vi "RydbergExpControl_2014.09.17_beta.vi"() -> ()   [LabVIEW 2013]
uses:
  rydberg_state_machine_states.ctl
  <userlib>/atmcd32d.llb/AcquisitionMode_mode typedef.ctl
  <userlib>/atmcd32d.llb/TriggerMode_mode typedef.ctl
  AndorCamera/camera_controls.ctl
  6704/6704_static_voltages_control.ctl
panel:
  in  "What To Change":enum16{"PulseBlaster", "Static Voltage"}(ring)
  in  "Trigger Snap Mode":bool
  in  "Shutdown Experiment":bool
  in  "Start Experiment":bool
  out "Started in trigger snap":bool=TRUE
  out "Waveform Chart":dbl(graph)
  in  "Count Number?":bool
  out "Number":dbl format="%^#_6g"
  out "OD":dbl[][](graph)
  out "Atom Closeup":dbl[][](graph)
  out "Atoms - BG":dbl[][](graph)
  out "Background Image":dbl[][](graph)
  out "Atom Image":dbl[][](graph)
  in  "Tab Control":T1(tab)
  out "Camera Ready":bool
  out "Exp Running":bool
  in  "PB Instruction Time To Change":i32
  in  "Static Channel To Change":i32
  in  "Step Size":dbl min=1e-06
  in  "Final Value":dbl
  in  "Initial Value":dbl
  in  "Instructions":T2(array[cluster])=[{"Instruct Data"=0, "Op Code"=0, "Flags"=[TRUE, FALSE, FALSE, FALSE, FALSE, FALSE, FALSE, FALSE, FALSE, FALSE, FALSE, FALSE, FALSE, FALSE, FALSE, FALSE, FALSE, FALSE, FALSE, FALSE, FALSE, FALSE, FALSE, FALSE], "Comments"="", "Time (s)"=0.1}, {"Instruct Data"=0, "Op Code"=0, "Flags"=[FALSE, FALSE, FALSE, FALSE, FALSE, FALSE, FALSE, FALSE, FALSE, FALSE, FALSE, FALSE, FALSE, FALSE, FALSE, FALSE, FALSE, FALSE, FALSE, FALSE, FALSE, FALSE, FALSE, FALSE], "Comments"="", "Time (s)"=0.1}, {"Instruct Data"=0, "Op Code"=0, "Flags"=[TRUE, FALSE, FALSE, FALSE, FALSE, FALSE, FALSE, FALSE, FALSE, FALSE, FALSE, FALSE, FALSE, FALSE, FALSE, FALSE, FALSE, FALSE, FALSE, FALSE, FALSE, FALSE, FALSE, FALSE], "Comments"="", "Time (s)"=0.1}, {"Instruct Data"=0, "Op Code"=6, "Flags"=[FALSE, FALSE, FALSE, FALSE, FALSE, FALSE, FALSE, FALSE, FALSE, FALSE, FALSE, FALSE, FALSE, FALSE, FALSE, FALSE, FALSE, FALSE, FALSE, FALSE, FALSE, FALSE, FALSE, FALSE], "Comments"="", "Time (s)"=0.1}] {"Time (s)" format="%.3p"; "Op Code" items=["Continue", "Stop", "Loop", "End Loop", "JSR", "RTS", "Branch", "Long Delay", "Wait"]}
  out "Scan Progress":dbl(slide) caption="Slide" scale=0.0..100.0
  out "Current Param Value":dbl
  in  "Parameter Nickname (no spaces)":string[](array[string])
  in  "Number of Parameters to Scan":i32=1 min=1
  in  "Channels to Change":dbl[](array[numeric])=[0.0, 0.0, 0.0]
  in  "Parameters to Change":enum16{"PulseBlaster", "Static Voltage"}[](array[ring])=[enum."Static Voltage", enum."Static Voltage", enum."Static Voltage"]
  in  "Step Sizes":dbl[](array[numeric])=[0.0, 0.0, 0.0]
  in  "Final Values":dbl[](array[numeric])=[0.0, 0.0, 0.0]
  in  "Initial Values":dbl[](array[numeric])
  in  "Scan Base Name":string
  in  "Raw_Data Folder":path
  out "Full Scan Name":string
  out "Camera Information":T3 {"VS Speed (us)" format="%.2f"}
  in  "Acquisition Parameters":T4={"Acquisition Mode"=enum."Kinetics", "Trigger Mode"=enum."External", "Frame \nTransfer"=FALSE, "Exposure Time (s)"=0.0001, "Accumulation Cycle Time (s)"=0.0, "# Accumulations"=1, "# Kinetics"=2, "Kinetic Cycle Time (s)"=0.0, "Horizontal Bin Size"=1, "Vertical Bin Size"=1} {"Vertical Bin Size" min=1; "Horizontal Bin Size" min=1; "Kinetic Cycle Time (s)" format="%.2f"; "# Kinetics" min=1; "# Accumulations" min=1; "Accumulation Cycle Time (s)" format="%.2f"; "Exposure Time (s)" format="%.2e"}
  out "Calcualted Times":T7 {"Kinetic" format="%.4f"; "Accumulate" format="%.4f"; "Exposure" format="%.4f"}
  in  "Red MOT 87 Inputs":T8={"Active Device"="6733_Red_87", "Active Channels"=[TRUE, FALSE, FALSE, FALSE, FALSE, FALSE, FALSE, FALSE], "Waveform Parameters"=[[{"Functional Form"=enum."Polynomial", "Start Voltage"=0.0, "End Voltage"=0.0, "Time"=0.0, "Degree"=1, "Sample Rate"=0.0}, {"Functional Form"=enum."Exponential", "Start Voltage"=0.0, "End Voltage"=0.0, "Time"=0.0, "Degree"=1, "Sample Rate"=0.0}, {"Functional Form"=enum."Exponential", "Start Voltage"=0.0, "End Voltage"=0.0, "Time"=0.0, "Degree"=1, "Sample Rate"=0.0}, {"Functional Form"=enum."Exponential", "Start Voltage"=0.0, "End Voltage"=0.0, "Time"=0.0, "Degree"=1, "Sample Rate"=0.0}, {"Functional Form"=enum."Exponential", "Start Voltage"=0.0, "End Voltage"=0.0, "Time"=0.0, "Degree"=1, "Sample Rate"=0.0}, {"Functional Form"=enum."Exponential", "Start Voltage"=0.0, "End Voltage"=0.0, "Time"=0.0, "Degree"=1, "Sample Rate"=0.0}], [{"Functional Form"=enum."Exponential", "Start Voltage"=0.0, "End Voltage"=0.0, "Time"=0.0, "Degree"=1, "Sample Rate"=0.0}, {"Functional Form"=enum."Exponential", "Start Voltage"=0.0, "End Voltage"=0.0, "Time"=0.0, "Degree"=1, "Sample Rate"=0.0}, {"Functional Form"=enum."Exponential", "Start Voltage"=0.0, "End Voltage"=0.0, "Time"=0.0, "Degree"=1, "Sample Rate"=0.0}, {"Functional Form"=enum."Exponential", "Start Voltage"=0.0, "End Voltage"=0.0, "Time"=0.0, "Degree"=1, "Sample Rate"=0.0}, {"Functional Form"=enum."Exponential", "Start Voltage"=0.0, "End Voltage"=0.0, "Time"=0.0, "Degree"=1, "Sample Rate"=0.0}, {"Functional Form"=enum."Exponential", "Start Voltage"=0.0, "End Voltage"=0.0, "Time"=0.0, "Degree"=1, "Sample Rate"=0.0}], [{"Functional Form"=enum."Exponential", "Start Voltage"=0.0, "End Voltage"=0.0, "Time"=0.0, "Degree"=1, "Sample Rate"=0.0}, {"Functional Form"=enum."Exponential", "Start Voltage"=0.0, "End Voltage"=0.0, "Time"=0.0, "Degree"=1, "Sample Rate"=0.0}, {"Functional Form"=enum."Exponential", "Start Voltage"=0.0, "End Voltage"=0.0, "Time"=0.0, "Degree"=1, "Sample Rate"=0.0}, {"Functional Form"=enum."Exponential", "Start Voltage"=0.0, "End Voltage"=0.0, "Time"=0.0, "Degree"=1, "Sample Rate"=0.0}, {"Functional Form"=enum."Exponential", "Start Voltage"=0.0, "End Voltage"=0.0, "Time"=0.0, "Degree"=1, "Sample Rate"=0.0}, {"Functional Form"=enum."Exponential", "Start Voltage"=0.0, "End Voltage"=0.0, "Time"=0.0, "Degree"=1, "Sample Rate"=0.0}], [{"Functional Form"=enum."Exponential", "Start Voltage"=0.0, "End Voltage"=0.0, "Time"=0.0, "Degree"=1, "Sample Rate"=0.0}, {"Functional Form"=enum."Exponential", "Start Voltage"=0.0, "End Voltage"=0.0, "Time"=0.0, "Degree"=1, "Sample Rate"=0.0}, {"Functional Form"=enum."Exponential", "Start Voltage"=0.0, "End Voltage"=0.0, "Time"=0.0, "Degree"=1, "Sample Rate"=0.0}, {"Functional Form"=enum."Exponential", "Start Voltage"=0.0, "End Voltage"=0.0, "Time"=0.0, "Degree"=1, "Sample Rate"=0.0}, {"Functional Form"=enum."Exponential", "Start Voltage"=0.0, "End Voltage"=0.0, "Time"=0.0, "Degree"=1, "Sample Rate"=0.0}, {"Functional Form"=enum."Exponential", "Start Voltage"=0.0, "End Voltage"=0.0, "Time"=0.0, "Degree"=1, "Sample Rate"=0.0}], [{"Functional Form"=enum."Exponential", "Start Voltage"=0.0, "End Voltage"=0.0, "Time"=0.0, "Degree"=1, "Sample Rate"=0.0}, {"Functional Form"=enum."Exponential", "Start Voltage"=0.0, "End Voltage"=0.0, "Time"=0.0, "Degree"=1, "Sample Rate"=0.0}, {"Functional Form"=enum."Exponential", "Start Voltage"=0.0, "End Voltage"=0.0, "Time"=0.0, "Degree"=1, "Sample Rate"=0.0}, {"Functional Form"=enum."Exponential", "Start Voltage"=0.0, "End Voltage"=0.0, "Time"=0.0, "Degree"=1, "Sample Rate"=0.0}, {"Functional Form"=enum."Exponential", "Start Voltage"=0.0, "End Voltage"=0.0, "Time"=0.0, "Degree"=1, "Sample Rate"=0.0}, {"Functional Form"=enum."Exponential", "Start Voltage"=0.0, "End Voltage"=0.0, "Time"=0.0, "Degree"=1, "Sample Rate"=0.0}], [{"Functional Form"=enum."Exponential", "Start Voltage"=0.0, "End Voltage"=0.0, "Time"=0.0, "Degree"=1, "Sample Rate"=0.0}, {"Functional Form"=enum."Exponential", "Start Voltage"=0.0, "End Voltage"=0.0, "Time"=0.0, "Degree"=1, "Sample Rate"=0.0}, {"Functional Form"=enum."Exponential", "Start Voltage"=0.0, "End Voltage"=0.0, "Time"=0.0, "Degree"=1, "Sample Rate"=0.0}, {"Functional Form"=enum."Exponential", "Start Voltage"=0.0, "End Voltage"=0.0, "Time"=0.0, "Degree"=1, "Sample Rate"=0.0}, {"Functional Form"=enum."Exponential", "Start Voltage"=0.0, "End Voltage"=0.0, "Time"=0.0, "Degree"=1, "Sample Rate"=0.0}, {"Functional Form"=enum."Exponential", "Start Voltage"=0.0, "End Voltage"=0.0, "Time"=0.0, "Degree"=1, "Sample Rate"=0.0}], [{"Functional Form"=enum."Exponential", "Start Voltage"=0.0, "End Voltage"=0.0, "Time"=0.0, "Degree"=1, "Sample Rate"=0.0}, {"Functional Form"=enum."Exponential", "Start Voltage"=0.0, "End Voltage"=0.0, "Time"=0.0, "Degree"=1, "Sample Rate"=0.0}, {"Functional Form"=enum."Exponential", "Start Voltage"=0.0, "End Voltage"=0.0, "Time"=0.0, "Degree"=1, "Sample Rate"=0.0}, {"Functional Form"=enum."Exponential", "Start Voltage"=0.0, "End Voltage"=0.0, "Time"=0.0, "Degree"=1, "Sample Rate"=0.0}, {"Functional Form"=enum."Exponential", "Start Voltage"=0.0, "End Voltage"=0.0, "Time"=0.0, "Degree"=1, "Sample Rate"=0.0}, {"Functional Form"=enum."Exponential", "Start Voltage"=0.0, "End Voltage"=0.0, "Time"=0.0, "Degree"=1, "Sample Rate"=0.0}], [{"Functional Form"=enum."Exponential", "Start Voltage"=0.0, "End Voltage"=0.0, "Time"=0.0, "Degree"=1, "Sample Rate"=0.0}, {"Functional Form"=enum."Exponential", "Start Voltage"=0.0, "End Voltage"=0.0, "Time"=0.0, "Degree"=1, "Sample Rate"=0.0}, {"Functional Form"=enum."Exponential", "Start Voltage"=0.0, "End Voltage"=0.0, "Time"=0.0, "Degree"=1, "Sample Rate"=0.0}, {"Functional Form"=enum."Exponential", "Start Voltage"=0.0, "End Voltage"=0.0, "Time"=0.0, "Degree"=1, "Sample Rate"=0.0}, {"Functional Form"=enum."Exponential", "Start Voltage"=0.0, "End Voltage"=0.0, "Time"=0.0, "Degree"=1, "Sample Rate"=0.0}, {"Functional Form"=enum."Exponential", "Start Voltage"=0.0, "End Voltage"=0.0, "Time"=0.0, "Degree"=1, "Sample Rate"=1.0}]], "Active Phases"=[TRUE, FALSE, FALSE, FALSE, FALSE, FALSE], "Phase Times"=[0.001], "Trigger Channel"="/6733_Red_87/PFI0"} {"Phase Times" format="%.0p"; "Waveform Parameters"."Degree" min=1}
  in  "6704 Static Voltage Settings":T9={"Device Name"="6704_Static", "Voltages"=[5.0, 0.0, 0.0, 0.0, 0.0, 0.0, 0.0, 0.0, 0.0, 0.0, 0.0, 0.0, 0.0, 0.0, 0.0, 0.0]}
  out "Andor Initialization Error Codes":T10
  out "Acq. Error Codes":T11
  out "Tree":string(tree)
  # "(1) 461 MOT beams"
  # "(2) Imaging AOM 1"
  # "(3) Imaging AOM 2"
  # "(4) Camera"
  # "(5) Zeeman shutter"
  # "(6) Repumper shutter"
  # "(7) 461 MOT coils"
  # "(8) 689 MOT coils"
  # "(9) 87 Sr Red MOT Trig"
  # "(10) ??? Shutter"
  # "(11) Red AOM"
  # "(12) Sat Abs Current Switch"
  # "(13) Zeeman MOSFET"
  # "1"
  # "2"
  # "3"
  # "4"
  # "5"
  # "6"
  # "7"
  # "8"
  # "9"
  # "10"
  # "11"
  # "12"
  # "13"
  # "14"
  # "15"
  # "16"
  # "17"
  # "18"
  # "19"
  # "20"
  # "21"
  # "22"
  # "23"
  # "24"
  # "Conversion formulae to be added"
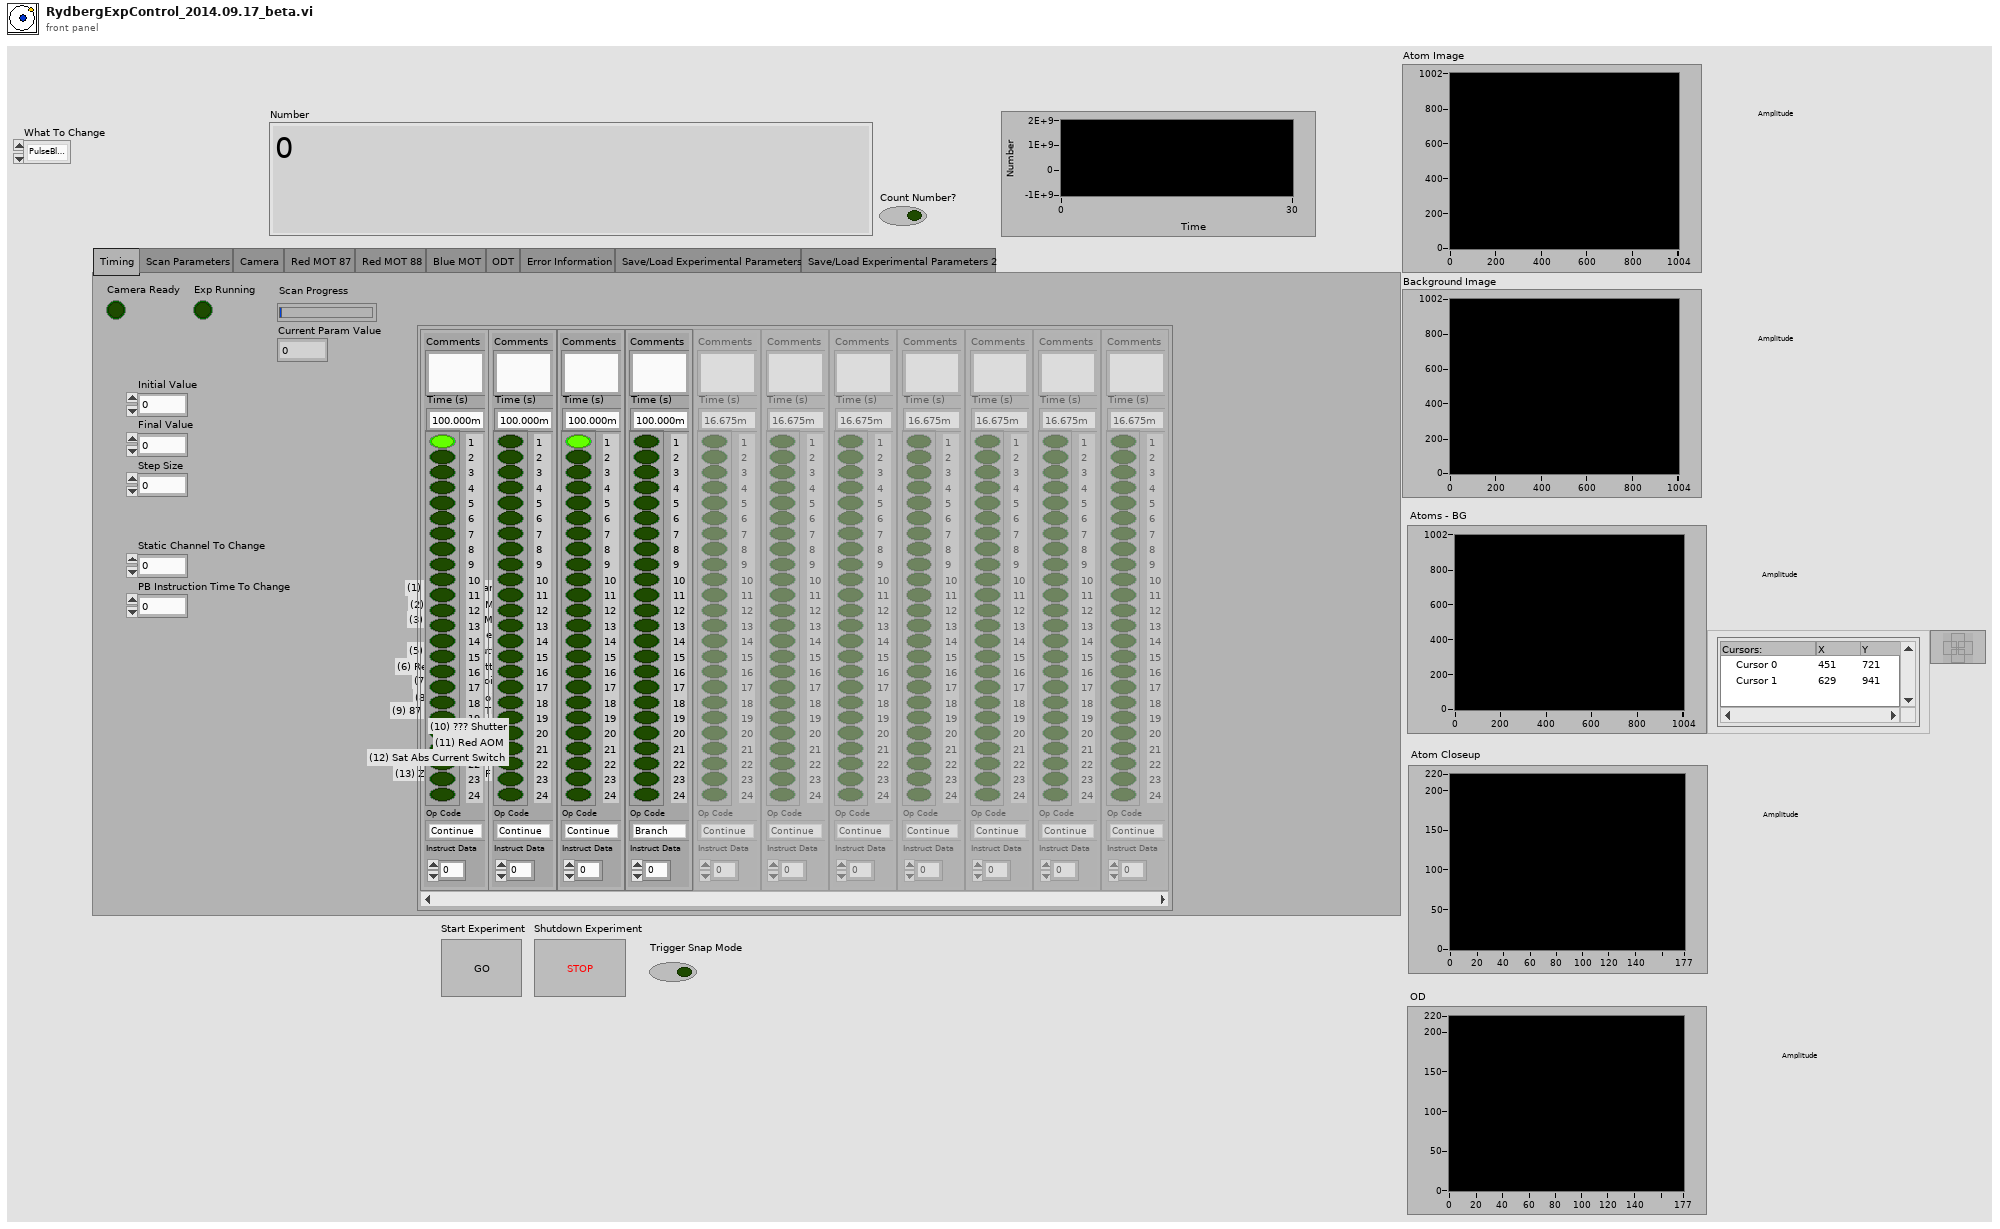
[diagram p1: front panel]
types:
  T1 = enum32{"Timing", "Scan Parameters", "Camera", "Red MOT 87", "Red MOT 88", "Blue MOT", "ODT", "Error Information", "Save/Load Experimental Parameters", "Save/Load Experimental Parameters 2"}
  T2 = cluster{"Instruct Data":i32, "Op Code":i32, "Flags":bool[], "Comments":string, "Time (s)":dbl}[]
  T3 = cluster{"xpixels":i32, "ypixels":i32, "# VS Speeds":i32, "VS Speed (us)":sgl, "Temperature Stable":bool, "Temperature (C)":i32}
  T4 = typedef "camera_controls.ctl" = cluster{"Acquisition Mode":T5, "Trigger Mode":T6, "Frame \nTransfer":bool, "Exposure Time (s)":sgl, "Accumulation Cycle Time (s)":sgl, "# Accumulations":i32, "# Kinetics":i32, "Kinetic Cycle Time (s)":sgl, "Horizontal Bin Size":i32, "Vertical Bin Size":i32}
  T5 = typedef "AcquisitionMode_mode typedef.ctl" = enum16{"Reserved (0)", "Single Scan", "Accumulate", "Kinetics", "Fast Kinetics", "Run Till Abort", "Reserved (6)", "Reserved (7)", "Reserved (8)", "Time Delayed Integration"}
  T6 = typedef "TriggerMode_mode typedef.ctl" = enum16{"Internal", "External", "N/A (2)", "N/A (3)", "N/A (4)", "N/A (5)", "External Start", "External Exposure (Bulb)", "N/A (8)", "External FVB EM", "Software", "N/A (11)", "External Charge Shifting"}
  T7 = cluster{"Exposure":sgl, "Accumulate":sgl, "Kinetic":sgl}
  T8 = cluster{"Active Device":string, "Active Channels":bool[], "Waveform Parameters":cluster{"Functional Form":enum16{"Polynomial", "Exponential"}, "Start Voltage":dbl, "End Voltage":dbl, "Time":dbl, "Degree":i8, "Sample Rate":dbl}[][], "Active Phases":bool[], "Phase Times":dbl[], "Trigger Channel":tag}
  T9 = typedef "6704_static_voltages_control.ctl" = cluster{"Device Name":string, "Voltages":dbl[]}
  T10 = cluster{"Initalize Error Code":u32, "GetDetector Error Code":u32, "Get#VSSpeeds Error Code":u32, "Set VS Speed Error":u32, "CoolerOn Error Code":u32, "GetTemperature Error Code":u32, "Shutdown Error Code":u32}
  T11 = cluster{"Set Acq. Mode Error":u32, "Set Trigger Mode Error":u32, "Set FT Error Code":u32, "Set Exposure Time Error Code":u32, "Set Accum Time Error":u32, "Set # Accum Error":u32, "Set # Kinetics Error":u32, "SetKinCycleTime Error":u32}
  T12 = typedef "rydberg_state_machine_states.ctl" = enum16{"Initialize", "Idle", "Experiment Running", "Trigger Snap Mode", "Scan Mode", "Load Experiment", "Shutdown"}
  T13 = cluster{"6704 Static Voltage Settings":T9, "Instructions":cluster{"Instruct Data":i32, "Op Code":i32, "Flags":bool[], "Comments":string, "Time (s)":dbl}[], "Red MOT 87 Inputs":cluster{"Active Device":string, "Active Channels":bool[], "Waveform Parameters":cluster{"Functional Form":enum16{"Polynomial", "Exponential"}, "Start Voltage":dbl, "End Voltage":dbl, "Time":dbl, "Degree":i8, "Sample Rate":dbl}[][], "Active Phases":bool[], "Phase Times":dbl[], "Trigger Channel":tag}}
  T14 = cluster{"Initial Values":refnum<vi>, "Channels to Change":refnum<vi>, "Final Values":refnum<vi>, "Step Sizes":refnum<vi>}
  T15 = typedef "LVCursorListTypeDef.ctl" = cluster{"Name":string, "Color":u32, "Style":u8, "Point Style":u8, "Name Visible":bool, "Allow Drag":bool, "Cursor Mode":u32, "Plot":i32, "Index":i32, "Position":cluster{"X":dbl, "Y":dbl}, "X Scale":u32, "Y Scale":u32, "Watch Plots":i32[], "Watch All Plots":bool, "Plot Area":i32, "Label Offset":cluster{"X":dbl, "Y":dbl}}[]
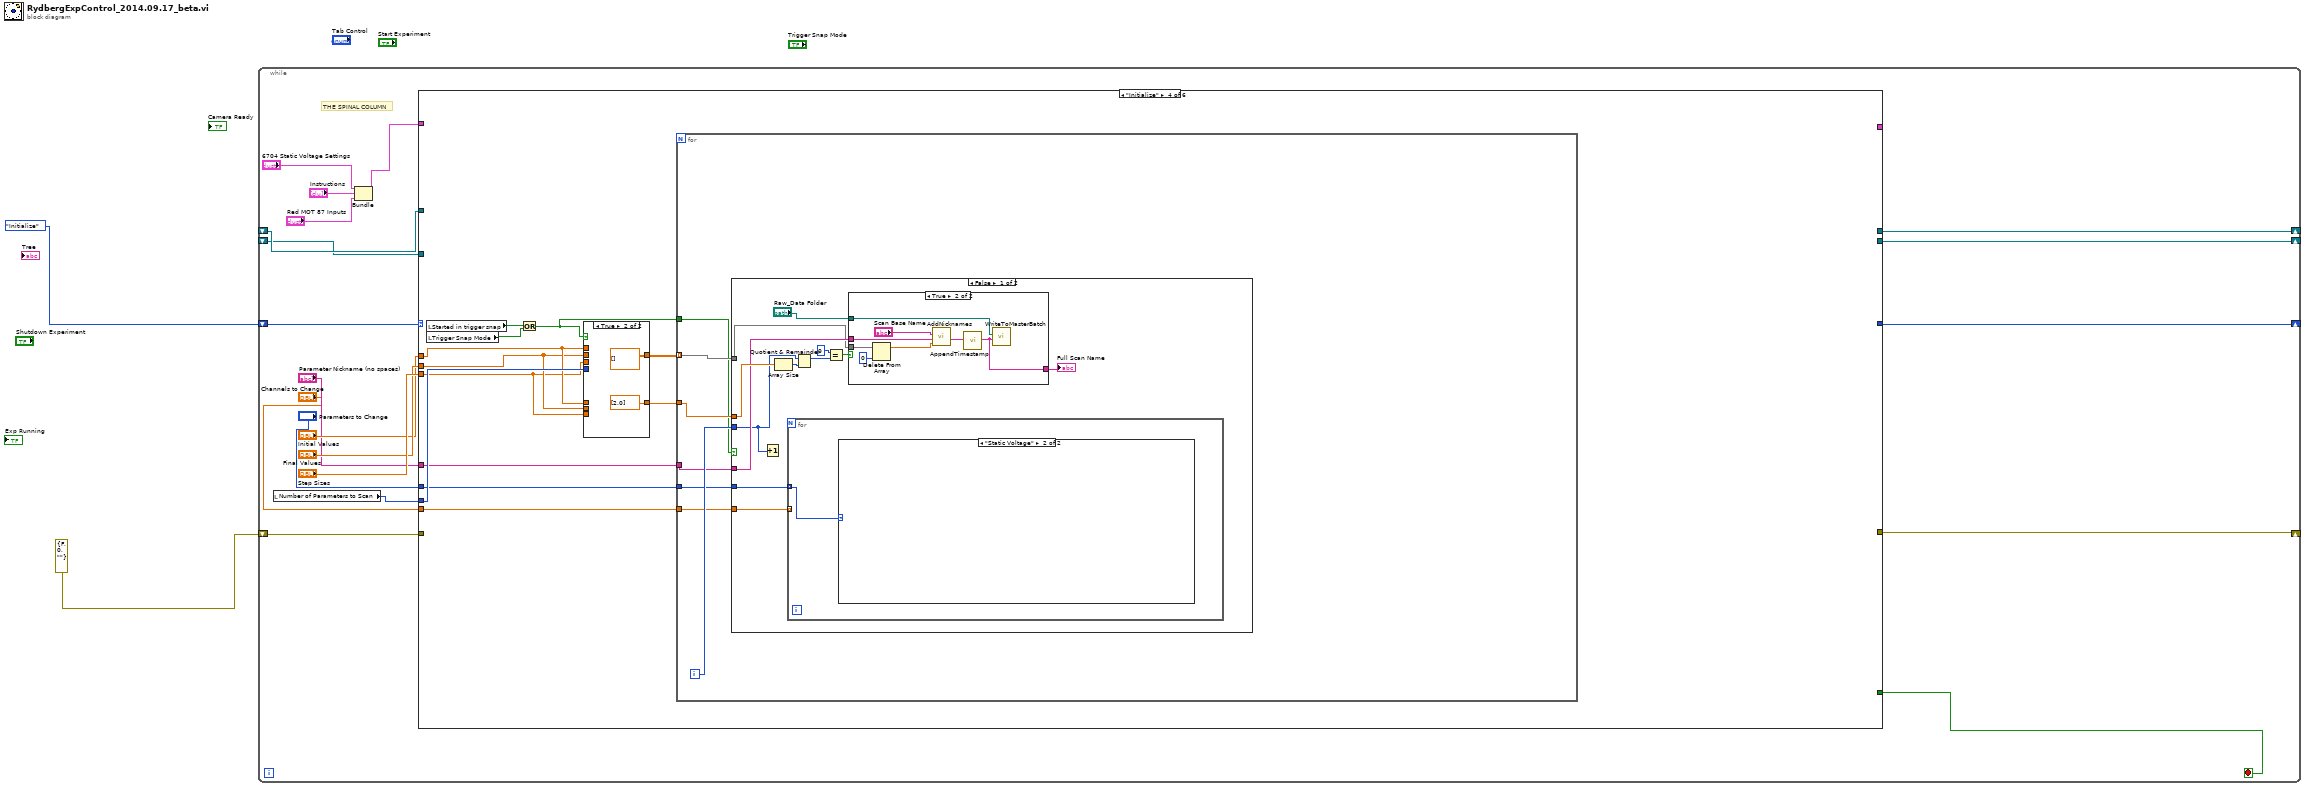
[diagram p0: block diagram]
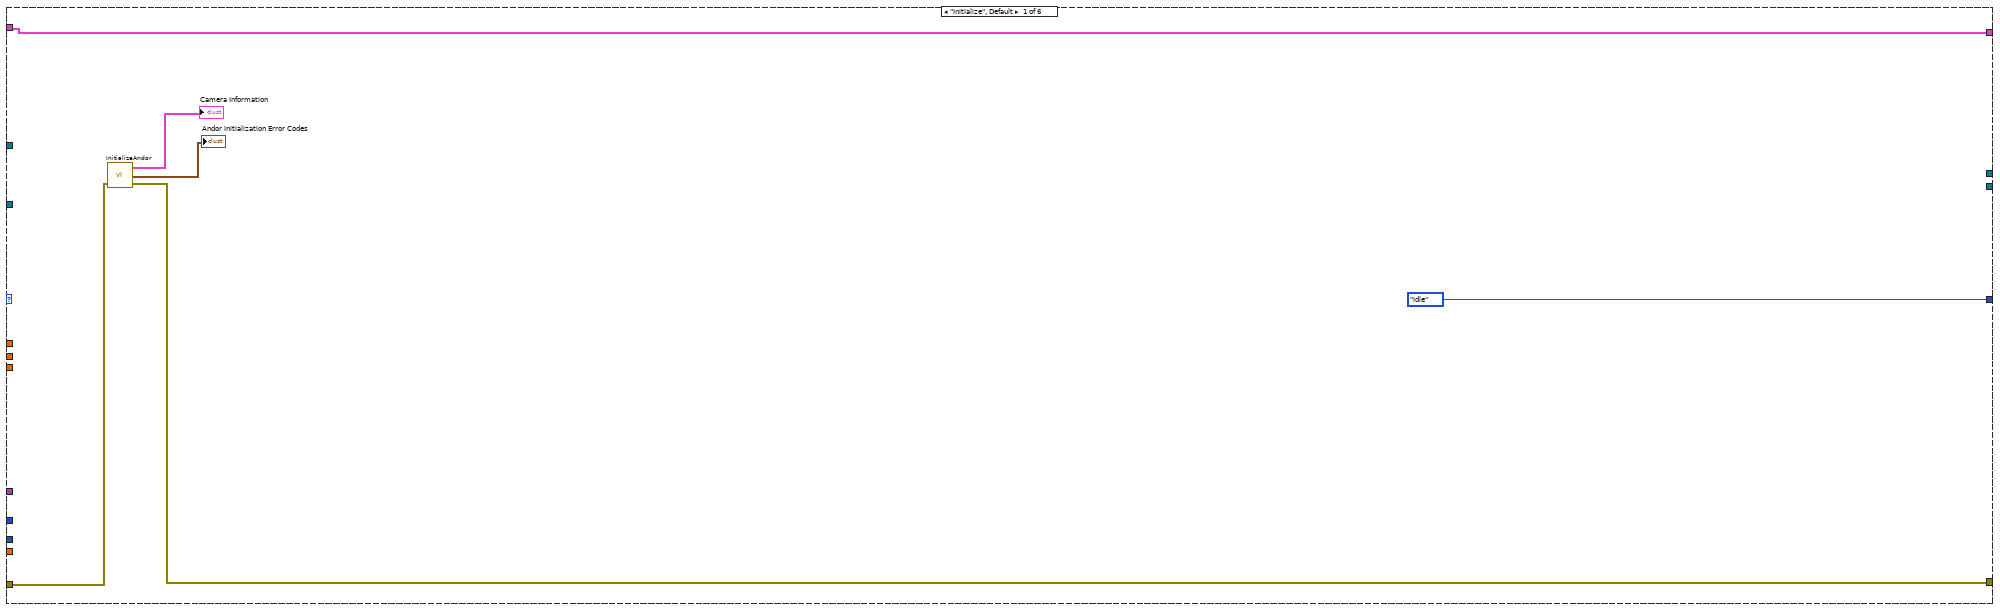
[diagram p2: hidden frame]
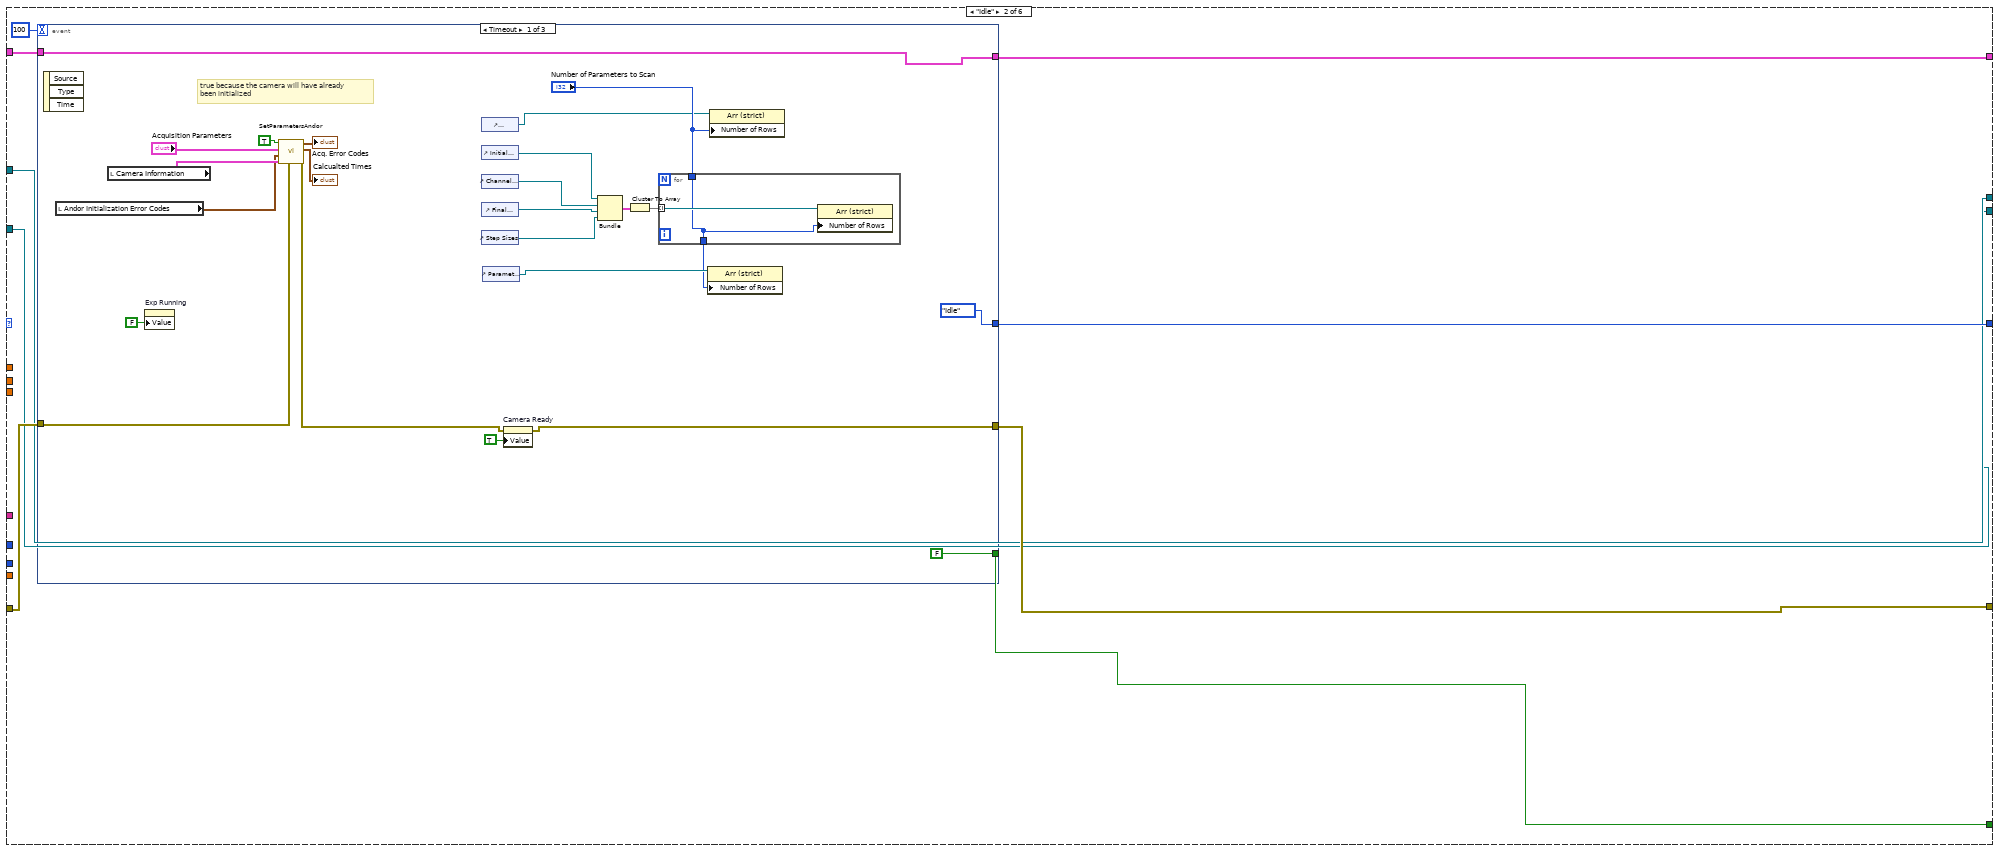
[diagram p3: hidden frame]
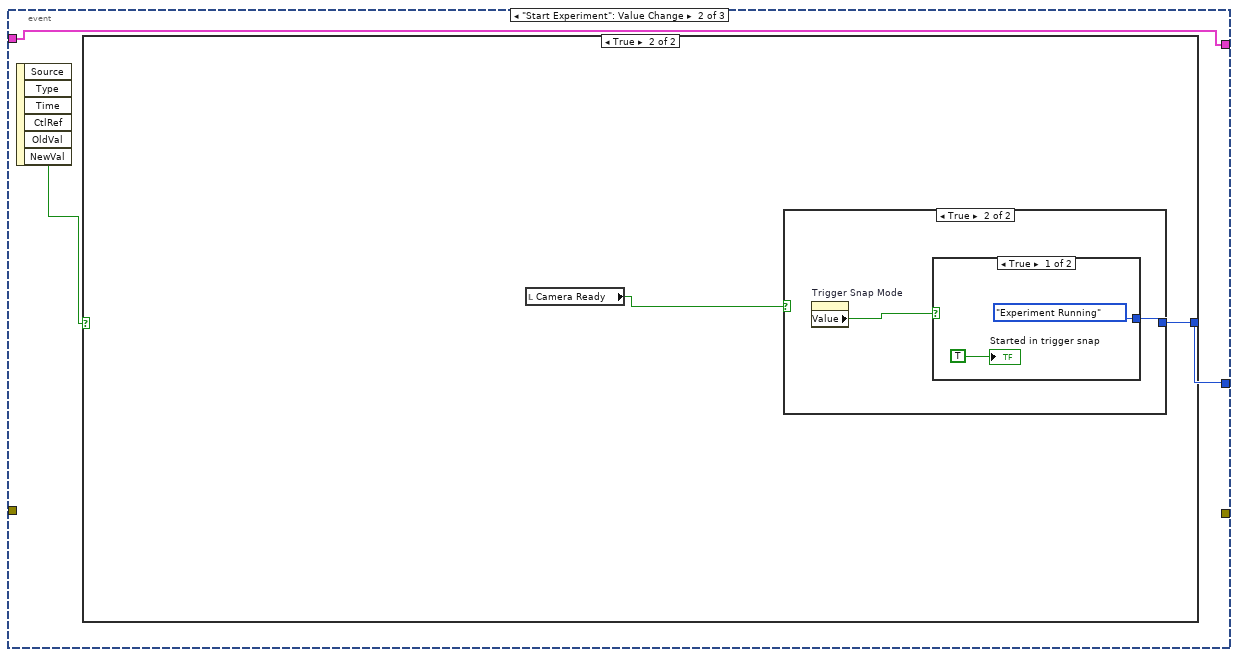
[diagram p4: hidden frame]
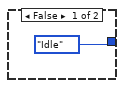
[diagram p5: hidden frame]
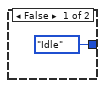
[diagram p6: hidden frame]
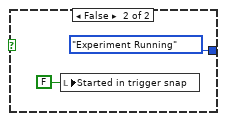
[diagram p7: hidden frame]
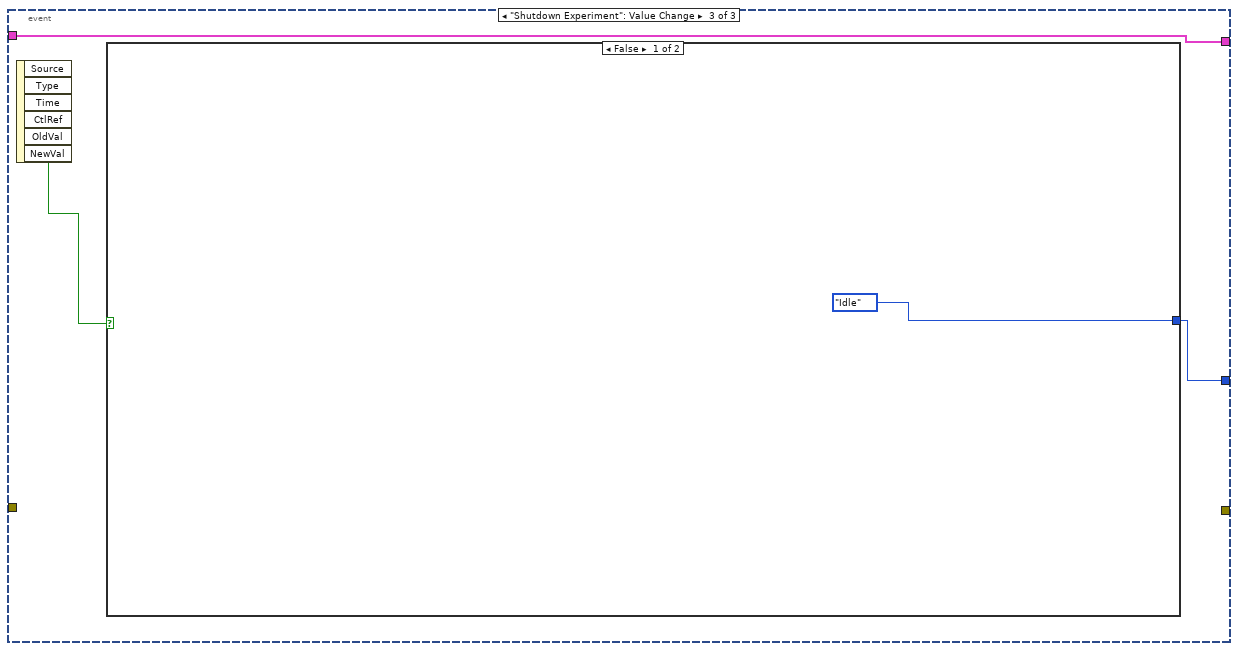
[diagram p8: hidden frame]
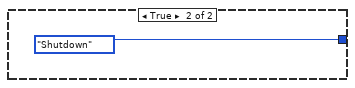
[diagram p9: hidden frame]
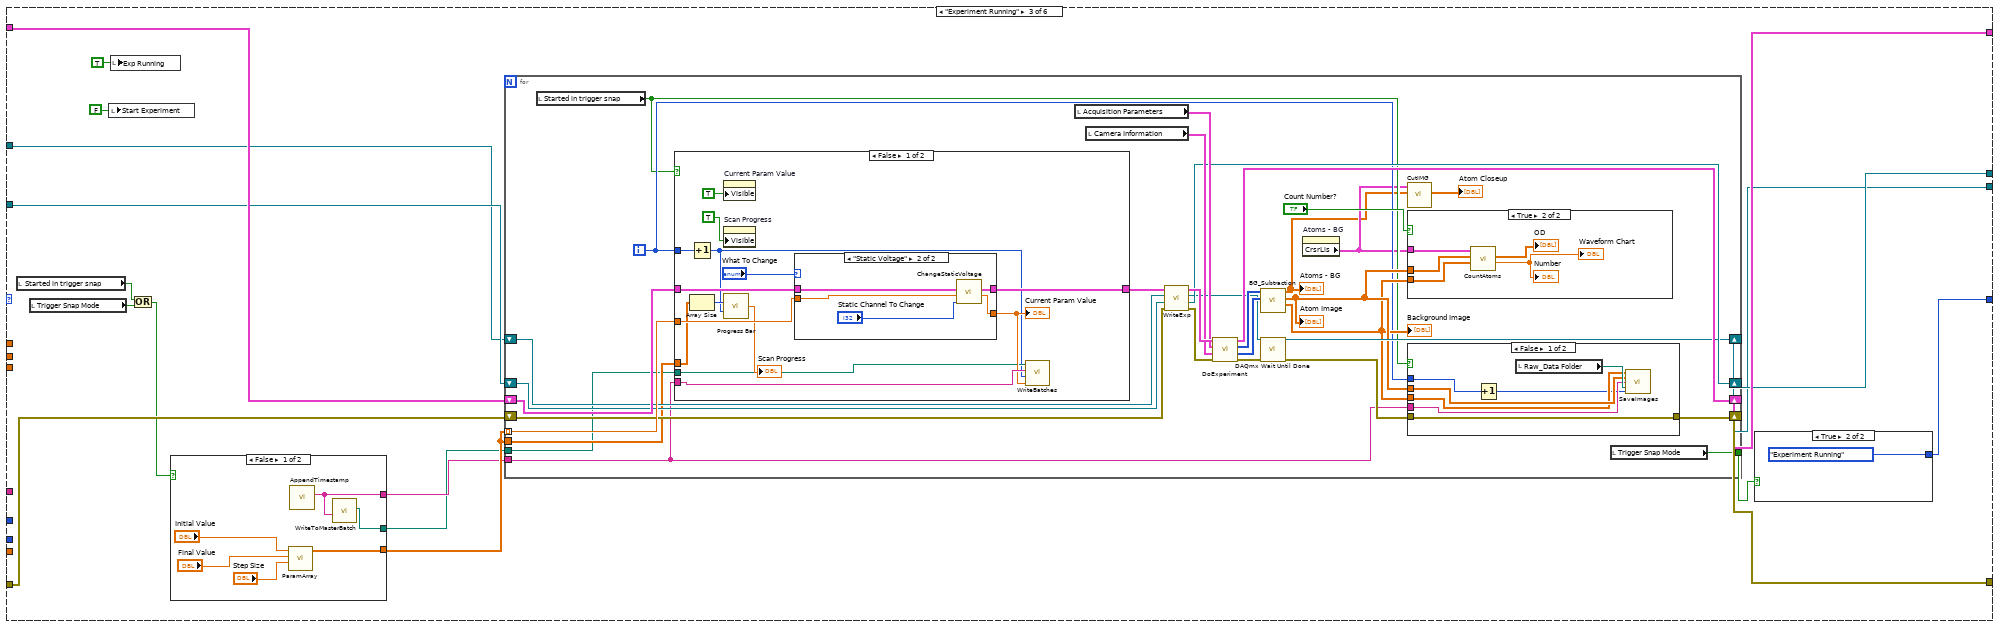
[diagram p10: hidden frame]
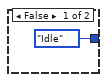
[diagram p11: hidden frame]
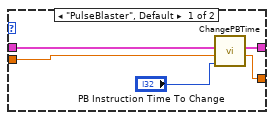
[diagram p14: hidden frame]
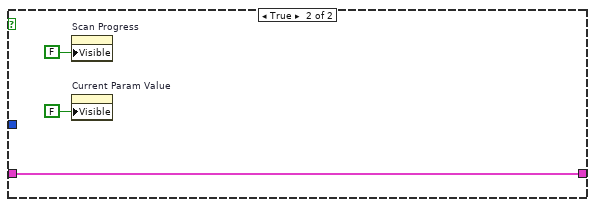
[diagram p15: hidden frame]
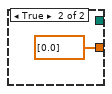
[diagram p16: hidden frame]
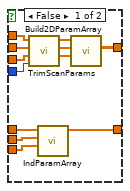
[diagram p20: hidden frame]
diagram:
  n1 = while {
    shift-right: [w19] -> _
    shift-left: rydberg_state_machine_states."Initialize" -> [w22]
    shift-right: [w20] -> _
    shift-left: errorcluster {"status"=FALSE, "code"=0, "source"=""} ("error constant") -> [w21]
    shift-right: [w13] -> _
    shift-left: _ -> [w12]
    shift-right: [w11] -> _
    shift-left: _ -> [w10]
    stop <- w18 stop-if-true
    # "THE SPINAL COLUMN"
    n2 = local read "Number of Parameters to Scan"() -> (w9:i32)
    n3 = Bundle("6704 Static Voltage Settings"="6704 Static Voltage Settings", "Instructions"="Instructions", "Red MOT 87 Inputs"="Red MOT 87 Inputs") -> (w14:T13)  [unwired: 1 in]
    n4 = case shown="\"Experiment Running2\"" w22 {
      tunnel: w21 -> [w28 w37 w97 _ _ w241]
      tunnel: [w25 w33 w95 _ _ w236] -> w20
      tunnel: [rydberg_state_machine_states."Idle" w35 w90 _ _ _] -> w19
      tunnel: [_ w34 _ _ _ TRUE] -> w18
      tunnel: [w23 w32 w92 _ w234 w238] -> _
      tunnel: w14 -> [w23 w31 w98 _ w234 w238]
      tunnel: [_ w30 w89 _ _ _] -> w13
      tunnel: w12 -> [_ w30 w86 _ _ _]
      tunnel: [_ w29 w88 _ _ _] -> w11
      tunnel: w10 -> [_ w29 w87 _ _ _]
      tunnel: w9 -> [_ _ _ w189 _ _]
      tunnel: "Step Sizes" -> [_ _ _ w185 _ _]
      tunnel: "Final Values" -> [_ _ _ w186 _ _]
      tunnel: "Initial Values" -> [_ _ _ w187 _ _]
      tunnel: "Parameter Nickname (no spaces)" -> [_ _ _ w182 _ _]
      tunnel: "Parameters to Change" -> [_ _ _ w181 _ _]
      tunnel: "Channels to Change" -> [_ _ _ w180 _ _]
      frame "Initialize", Default {
        n5 = call "InitializeAndor.vi"("Error In"=w28) -> ("error out"=w25:errorcluster, "Andor Initialization Error Codes"=→"Andor Initialization Error Codes":T10, "Camera Information"=→"Camera Information":T3)  [unwired: 2 in]
      }
      frame "Idle" {
        n6 = event shown="[0] Timeout" {
          selector: _ -> [_ _ _]
          dyn-events: _ -> [_ _ _]
          timeout: 100 -> [_ _ _]
          tunnel: w37 -> [w55 _ _]
          tunnel: [rydberg_state_machine_states."Idle" w65 w78] -> w35
          tunnel: [FALSE _ _] -> w34
          tunnel: [w49 _ _] -> w33
          tunnel: [w52 w64 w77] -> w32
          tunnel: w31 -> [w52 w64 w77]
          event Timeout {
            # "true because the camera will have already\nbeen initialized"
            n7 = event-data() -> ()  [unwired: 1 in, 3 out]
            n8 = local read "Andor Initialization Error Codes"() -> (w54:T10)
            n9 = local read "Camera Information"() -> (w57:T3)
            n10 = property on="Exp Running" class="Bool (strict)"("Value"=FALSE ("Exp Running")) -> ()  [unwired: 2 in, 2 out]
            n11 = call "SetParametersAndor.vi"("Error In"=w55, "Camera Information"=w57, "Andor Initialization Error Codes"=w54, "Acquisition Parameters"="Acquisition Parameters", "Pre Initialized?"=TRUE) -> ("error out"=w50:errorcluster, "Calcualted Times"=→"Calcualted Times":T7, "Acq. Error Codes"=→"Acq. Error Codes":T11)  [unwired: 4 in]
            n12 = control-ref of="Parameters to Change"() -> (w40:refnum<vi>)
            n13 = control-ref of="Initial Values"() -> (w47:refnum<vi>)
            n14 = control-ref of="Channels to Change"() -> (w46:refnum<vi>)
            n15 = control-ref of="Final Values"() -> (w45:refnum<vi>)
            n16 = control-ref of="Step Sizes"() -> (w44:refnum<vi>)
            n17 = control-ref of="Parameter Nickname (no spaces)"() -> (w39:refnum<vi>)
            n18 = property on="Camera Ready" class="Bool (strict)"(error in=w50, "Value"=TRUE ("Camera Ready")) -> (error out=w49:errorcluster)  [unwired: 1 in, 1 out]
            n19 = Bundle("Initial Values"=w47, "Channels to Change"=w46, "Final Values"=w45, "Step Sizes"=w44) -> (w43:T14)  [unwired: 1 in]
            n20 = Cluster To Array(cluster=w43) -> (array=w42:refnum<vi>[])
            n21 = for {
              tunnel: w42 -> [w63] mode=indexing
              tunnel: "Number of Parameters to Scan" -> [w62]
              tunnel: [w62] -> w38
              n22 = property class="Arr (strict)"(reference=w63, "Number of Rows"=w62) -> ()  [unwired: 1 in, 2 out]
            }
            n23 = property class="Arr (strict)"(reference=w39, "Number of Rows"=w38) -> ()  [unwired: 1 in, 2 out]
            n24 = property class="Arr (strict)"(reference=w40, "Number of Rows"="Number of Parameters to Scan") -> ()  [unwired: 1 in, 2 out]
          }
          event "Start Experiment": Value Change {
            n25 = event-data() -> ("NewVal"=w66:bool)  [unwired: 1 in, 5 out]
            n26 = case shown="True" w66 {
              tunnel: [rydberg_state_machine_states."Idle" w69] -> w65
              frame False {
              }
              frame True {
                n27 = local read "Camera Ready"() -> (w68:bool)
                n28 = case shown="True" w68 {
                  tunnel: [rydberg_state_machine_states."Idle" w72] -> w69
                  frame False {
                  }
                  frame True {
                    n29 = property on="Trigger Snap Mode" class="Bool (strict)"() -> ("Value"=w71:bool)  [unwired: 2 in, 2 out]
                    n30 = case shown="True" w71 {
                      tunnel: [rydberg_state_machine_states."Experiment Running" rydberg_state_machine_states."Experiment Running"] -> w72
                      frame True {
                        "Started in trigger snap" <- TRUE
                      }
                      frame False {
                        n31 = local write "Started in trigger snap"(FALSE ("Started in trigger snap")) -> ()
                      }
                    }
                  }
                }
              }
            }
          }
          event "Shutdown Experiment": Value Change {
            n32 = event-data() -> ("NewVal"=w79:bool)  [unwired: 1 in, 5 out]
            n33 = case shown="False" w79 {
              tunnel: [rydberg_state_machine_states."Idle" rydberg_state_machine_states."Shutdown"] -> w78
              frame False {
              }
              frame True {
              }
            }
          }
        }
      }
      frame "Experiment Running" {
        n34 = local read "Started in trigger snap"() -> (w83:bool)
        n35 = local read "Trigger Snap Mode"() -> (w84:bool)
        n36 = local write "Start Experiment"(FALSE ("Start Experiment")) -> ()
        n37 = local write "Exp Running"(TRUE ("Exp Running")) -> ()
        n38 = Or(x=w83, y=w84) -> (x .or. y?=w82:bool)
        n39 = case shown="False" w82 {
          tunnel: [w175 dbl[] [0.0]] -> w96
          tunnel: [w174 _] -> w94
          tunnel: [w173 _] -> w93
          frame False {
            n40 = call "ParamArray.vi"("Step Size"="Step Size", "Final Value"="Final Value", "Initial Value"="Initial Value") -> ("Array"=w175:dbl[])  [unwired: 8 in]
            n41 = call "AppendTimestamp.vi"() -> ("String 2"=w174:string)  [unwired: 11 in]
            n42 = call "WriteToMasterBatch.vi"("Scan name"=w174) -> ("Raw_Data Folder"=w173:path)  [unwired: 10 in]
          }
          frame True {
          }
        }
        n43 = for {
          shift-right: [w121] -> w92
          shift-left: w98 -> [w132]
          tunnel: w96 -> [w131] mode=indexing
          shift-right: [w114] -> w89
          shift-left: w86 -> [w120]
          shift-right: [w118] -> w88
          shift-left: w87 -> [w119]
          tunnel: w96 -> [w117]
          shift-right: [w111] -> w95
          shift-left: w97 -> [w129]
          tunnel: w94 -> [w107]
          tunnel: w93 -> [w113]
          tunnel: [w106] -> w91
          i -> [w108]
          n44 = local read "Started in trigger snap"() -> (w105:bool)
          n45 = case shown="False" w105 {
            tunnel: w132 -> [w159 w172]
            tunnel: w131 -> [w158 _]
            tunnel: [w157 w172] -> w130
            tunnel: w108 -> [w148 _]
            tunnel: w117 -> [w156 _]
            tunnel: w107 -> [w153 _]
            tunnel: w113 -> [w151 _]
            frame False {
              n46 = Increment(x=w148) -> (x+1=w147:i32)
              n47 = Array Size(array=w156) -> (size(s)=w155:i32)
              n48 = property on="Current Param Value" class="DigNum (strict)"("Visible"=TRUE) -> ()  [unwired: 2 in, 2 out]
              n49 = property on="Scan Progress" class="Slide (strict)"("Visible"=TRUE) -> ()  [unwired: 2 in, 2 out]
              n50 = call "Progress Bar.vi"("Total Number"=w155, "Current Number"=w147) -> ("Scan Progress"=→"Scan Progress":dbl)  [unwired: 13 in]
              n51 = case shown="\"Static Voltage\"" "What To Change" {
                tunnel: w159 -> [w164 w169]
                tunnel: w158 -> [w161 w167]
                tunnel: [w163 w166] -> w157
                tunnel: [w160 w165] -> w152
                frame "PulseBlaster", Default {
                  n52 = call "ChangePBTime.vi"("Instruction to change"="PB Instruction Time To Change", "Time"=w161, "Input parameters"=w164) -> ("Time out"=w160:dbl, "output parameters"=w163:T13)  [unwired: 7 in]
                }
                frame "Static Voltage" {
                  n53 = call "ChangeStaticVoltage.vi"("Channel to change"="Static Channel To Change", "Voltage"=w167, "Parameters input"=w169) -> ("Voltage out"=w165:dbl, "Parameters Output"=w166:T13)  [unwired: 7 in]
                }
              }
              "Current Param Value" <- w152
              n54 = call "WriteBatches.vi"("Variable Parameter Value"=w152, "Image Number"=w147, "String"=w153, "Raw Data Folder"=w151) -> ()  [unwired: 8 in]
            }
            frame True {
              n55 = property on="Scan Progress" class="Slide (strict)"("Visible"=FALSE) -> ()  [unwired: 2 in, 2 out]
              n56 = property on="Current Param Value" class="DigNum (strict)"("Visible"=FALSE) -> ()  [unwired: 2 in, 2 out]
            }
          }
          n57 = local read "Acquisition Parameters"() -> (w126:T4)
          n58 = local read "Camera Information"() -> (w127:T3)
          n59 = call "WriteExp.vi"("error in (no error)"=w129, "Control Task In"=w119, "Waveform Task In"=w120, "Experimental Control Cluster In"=w130) -> ("error out"=w125:errorcluster, "waveform task out"=w118:refnum<k21>, "counter task out"=w116:refnum<k21>, "Experimental Control Cluster Out"=w128:T13)  [unwired: 4 in]
          n60 = call "DoExperiment.vi"("Error In"=w125, "Camera Information 2"=w127, "Acquisition Parameters"=w126, "output cluster"=w128) -> ("error out"=w115:errorcluster, "Background Image"=w124:i32[][], "Atom Image"=w123:i32[][], "output cluster 2"=w121:T13)  [unwired: 4 in]
          n61 = call "BG_Subtraction.vi"("Background Image"=w124, "Atom Image"=w123) -> ("Background Image Out"=w109:dbl[][], "Atom Image Out"=w110:dbl[][], "Atoms - BG"=w103:dbl[][])  [unwired: 7 in]
          "Background Image" <- w109
          "Atom Image" <- w110
          "Atoms - BG" <- w103
          n62 = call <vilib>:"DAQmx Wait Until Done.vi"("task/channels in"=w116, "error in"=w115) -> ("task out"=w114:refnum<k21>, "error out"=w112:errorcluster)  [unwired: 12 in]
          n63 = property on="Atoms - BG" class="IntGraph (strict)"() -> ("CrsrLis"=w104:T15)  [unwired: 2 in, 2 out]
          n64 = call "CutIMG.vi"("Full Image In"=w103, "Cursor List"=w104) -> ("Cut Image Out"=→"Atom Closeup":dbl[][])  [unwired: 9 in]
          n65 = case shown="True" "Count Number?" {
            tunnel: w104 -> [_ w145]
            tunnel: w110 -> [_ w144]
            tunnel: w109 -> [_ w143]
            frame False {
            }
            frame True {
              n66 = call "CountAtoms.vi"("Background Image"=w143, "Atom Image"=w144, "Cursor List"=w145) -> ("Number"=→"Waveform Chart" →"Number":dbl, "OD"=→"OD":dbl[][])  [unwired: 7 in]
            }
          }
          n67 = case shown="False" w105 {
            tunnel: [w139 w140] -> w111
            tunnel: w112 -> [w139 w140]
            tunnel: w110 -> [w137 _]
            tunnel: w109 -> [w136 _]
            tunnel: w108 -> [w134 _]
            tunnel: w107 -> [w135 _]
            frame False {
              n68 = Increment(x=w134) -> (x+1=w133:i32)
              n69 = local read "Raw_Data Folder"() -> (w138:path)
              n70 = call "SaveImages.vi"("Background Image"=w136, "Atoms Image"=w137, "Base Filename"=w135, "Raw Data Path"=w138, "ImageNumber"=w133) -> ()  [unwired: 9 in, 2 out]
            }
            frame True {
            }
          }
          n71 = local read "Trigger Snap Mode"() -> (w106:bool)
        }
        n72 = case shown="True" w91 {
          tunnel: [rydberg_state_machine_states."Idle" rydberg_state_machine_states."Experiment Running"] -> w90
          frame False {
          }
          frame True {
          }
        }
      }
      frame "Initialize" {
        n73 = local read "Started in trigger snap"() -> (w190:bool)
        n74 = local read "Trigger Snap Mode"() -> (w191:bool)
        n75 = Or(x=w190, y=w191) -> (x .or. y?=w183:bool)
        n76 = case shown="True" w183 {
          tunnel: w189 -> [w231 _]
          tunnel: w185 -> [w230 _]
          tunnel: w186 -> [w229 _]
          tunnel: w187 -> [w228 _]
          tunnel: [w224 dbl[][] [] ("Parameter Array")] -> w188
          tunnel: w187 -> [w223 _]
          tunnel: w186 -> [w222 _]
          tunnel: w185 -> [w221 _]
          tunnel: [w220 dbl[] [2.0] ("Array")] -> w184
          frame False {
            n77 = call "TrimScanParams.vi"("Parameters to change"=w231, "Step Sizes"=w230, "Final Values"=w229, "Initial Values"=w228) -> ("Step Sizes Out"=w225:dbl[], "Final Values Out"=w226:dbl[], "Initial Values Out"=w227:dbl[])  [unwired: 5 in]
            n78 = call "IndParamArray.vi"("Step Sizes"=w221, "Final Values"=w222, "Initial Values"=w223) -> ("Array"=w220:dbl[])  [unwired: 8 in]
            n79 = call "Build2DParamArray.vi"("Step Sizes"=w225, "Final Values"=w226, "Initial Values"=w227) -> ("Parameter Array"=w224:dbl[][])  [unwired: 8 in]
          }
          frame True {
          }
        }
        n80 = for {
          tunnel: w188 -> [w195] mode=indexing
          tunnel: w184 -> [w198]
          tunnel: w183 -> [w194]
          tunnel: w182 -> [w196]
          tunnel: w181 -> [w193]
          tunnel: w180 -> [w192]
          i -> [w197]
          n81 = case shown="False" w194 {
            tunnel: w198 -> [w210 _]
            tunnel: w197 -> [w199 _]
            tunnel: w196 -> [w206 _]
            tunnel: w195 -> [w205 _]
            tunnel: w193 -> [w203 _]
            tunnel: w192 -> [w202 _]
            frame False {
              n82 = Increment(x=w199) -> ()  [unwired: 1 out]
              n83 = Array Size(array=w210) -> (size(s)=w209:i32)
              n84 = for {
                tunnel: w203 -> [w211] mode=indexing
                tunnel: w202 -> [_] mode=indexing
                n85 = case shown="\"Static Voltage\"" w211 {
                  frame "PulseBlaster", Default {
                  }
                  frame "Static Voltage" {
                  }
                }
              }
              n86 = Quotient & Remainder(x=w199, y=w209) -> (x-y*floor(x/y)=w208:i32)  [unwired: 1 out]
              n87 = Equal?(x=0, y=w208) -> (x = y?=w204:bool)
              n88 = case shown="True" w204 {
                tunnel: w206 -> [_ w219]
                tunnel: w205 -> [_ w218]
                tunnel: "Raw_Data Folder" -> [_ w213]
                tunnel: [_ w212] -> w200
                frame False {
                }
                frame True {
                  n89 = Delete From Array(array=w218, index=0) -> (array with subset deleted=w215:dbl[])  [unwired: 1 in, 1 out]
                  n90 = call "AddNicknames.vi"("Values"=w215, "Nicknames"=w219, "Base Name"="Scan Base Name") -> ("Name Out"=w214:string)  [unwired: 8 in]
                  n91 = call "AppendTimestamp.vi"("String"=w214) -> ("String 2"=w212:string)  [unwired: 10 in]
                  n92 = call "WriteToMasterBatch.vi"("Scan name"=w212, "Raw_Data Folder"=w213) -> ()  [unwired: 10 in]
                }
              }
              "Full Scan Name" <- w200
            }
            frame True {
            }
          }
        }
      }
      frame "Load Experiment" {
      }
      frame "Shutdown" {
        n93 = call <userlib>:"ShutDown.vi"("error in (no error)"=w241) -> ("error out"=w237:errorcluster)  [unwired: 1 in, 1 out]
        n94 = property on="Camera Ready" class="Bool (strict)"(error in=w237, "Value"=FALSE ("Camera Ready")) -> (error out=w236:errorcluster)  [unwired: 1 in, 1 out]
        n95 = local write "Shutdown Experiment"(FALSE ("Shutdown Experiment")) -> ()
      }
    }
  }
